vi "Initialize.vi"(8 "error in (no error)":errorcluster, 11 "HSDIO in":refnum<class "HSDIO.lvclass">) -> (0 "error out":errorcluster, 3 "HSDIO out":refnum<class "HSDIO.lvclass">)   [LabVIEW 2013, in "HSDIO.lvclass"]
uses:
  HSDIO.lvclass
  HSDIO.lvclass/HSDIO.ctl
  <instrlib>/niHSDIO/niHSDIO.llb/niHSDIO_ctl Sample Clock Source Values (ComboBox).ctl
  <instrlib>/niHSDIO/niHSDIO.llb/niHSDIO_ctl Generation Mode Values (Ring).ctl
  Globals.vi
  <instrlib>/niHSDIO/niHSDIO.llb/niHSDIO Configure Initial State (String).vi
  <instrlib>/niHSDIO/niHSDIO.llb/niHSDIO Configure Idle State (String).vi
  <instrlib>/niHSDIO/niHSDIO.llb/niHSDIO Configure Digital Edge Script Trigger.vi
  <instrlib>/niHSDIO/niHSDIO.llb/niHSDIO Configure Digital Level Script Trigger.vi
  <instrlib>/niHSDIO/niHSDIO.llb/niHSDIO Configure Digital Edge Start Trigger.vi
panel:
  out "HSDIO Settings.Idle State":string
  out "HSDIO Settings.Inital State":string
  out "HSDIO Status.Channel List":string
  out "instrument handle out":refnum<k15>
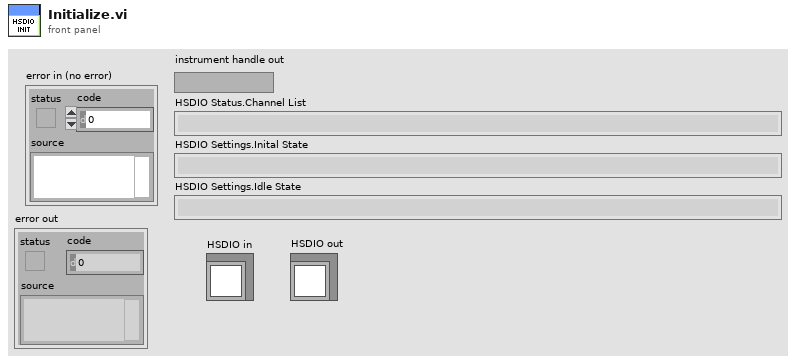
[diagram p1: front panel]
types:
  T1 = typedef "niHSDIO_ctl Sample Clock Source Values (ComboBox).ctl" = string
  T2 = typedef "niHSDIO_ctl Generation Mode Values (Ring).ctl" = i32
  T3 = typedef "niHSDIO_ctl Trigger Source Values (Ring).ctl" = string
  T4 = typedef "niHSDIO_ctl Trigger DigEdge - Edge Values (Ring).ctl" = i32
  T5 = cluster{"Wait for start trigger?":bool, "source (PFI 0)":T3, "edge (rising)":T4, "description":string}
  T6 = typedef "niHSDIO_ctl Trigger Script - trigID Values (Ring).ctl" = string
  T7 = typedef "niHSDIO_ctl Trigger DigLvl - Level Values (Ring).ctl" = i32
  T8 = cluster{"trigger id (script trigger 0)":T6, "source (PFI 0)":T3, "Trigger Type":enum32{"Edge", "Level"}, "edge":T4, "level":T7}[]
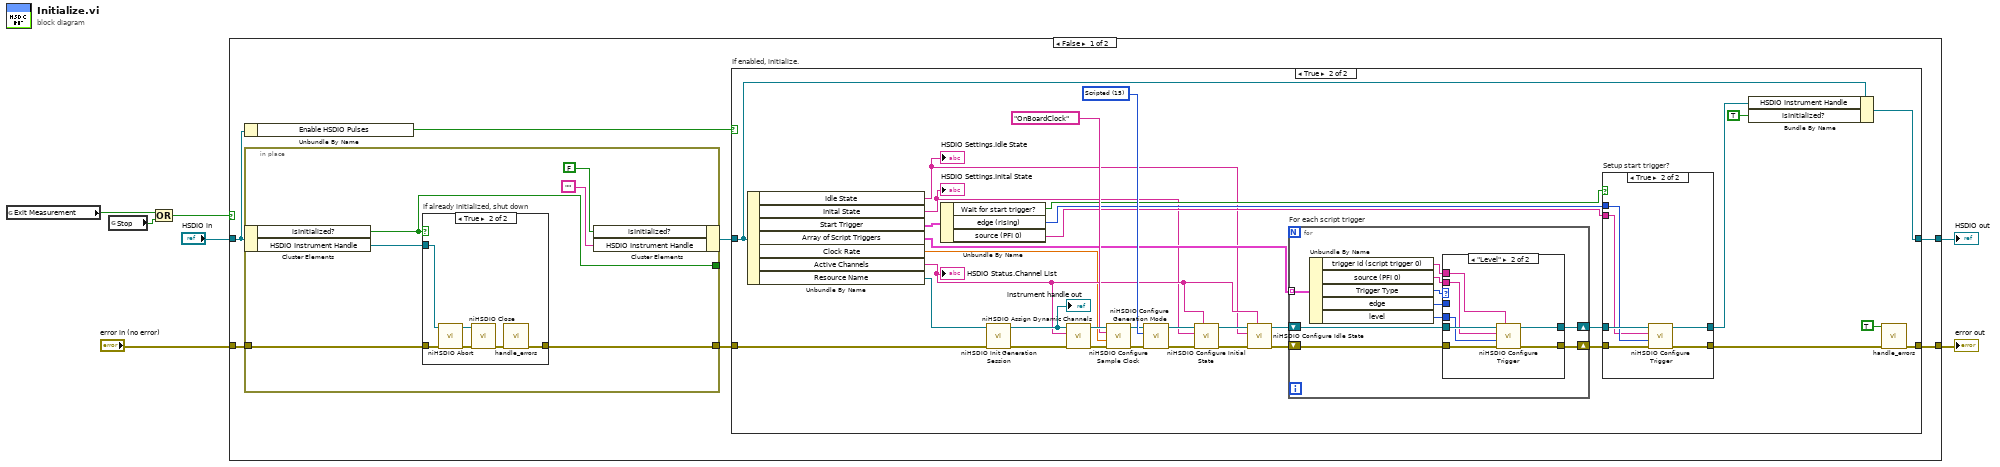
[diagram p0: block diagram]
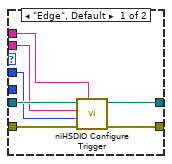
[diagram p4: hidden frame]
diagram:
  n1 = global read "Globals.vi" "Exit Measurement"() -> (w4:bool)
  n2 = global read "Globals.vi" "Stop"() -> (w3:bool)
  n3 = Or(x=w4, y=w3) -> (x .or. y?=w2:bool)
  n4 = case shown="False" w2 {
    tunnel: [w8 w96] -> w7
    tunnel: [w13 w97] -> w5
    tunnel: "HSDIO in" -> [w12 w97]
    tunnel: "error in (no error)" -> [w10 w96]
    frame False {
      n5 = Unbundle By Name(w12) -> ("Enable HSDIO Pulses"=w14:bool)
      n6 = in-place {
        in-place-border: [w17] -> _
        in-place-border: w10 -> [w20]
        in-place-border: [w19] -> w9
        n7 = in-place-cluster #1(w12) -> ("isInitialized?"=w17:bool, "HSDIO Instrument Handle"=w18:refnum<k15>)
        n8 = case "if already initialized, shut down" shown="True" w17 {
          tunnel: w20 -> [w21 w26]
          tunnel: [w21 w23] -> w19
          tunnel: w18 -> [_ w22]
          frame False {
          }
          frame True {
            n9 = call <instrlib>:"niHSDIO Abort.vi"("error in (no error)"=w26, "instrument handle"=w22) -> ("error out"=w25:errorcluster, "instrument handle out"=w27:refnum<k15>)  [unwired: 8 in]
            n10 = call <instrlib>:"niHSDIO Close.vi"("error in (no error)"=w25, "instrument handle"=w27) -> ("error out"=w24:errorcluster)  [unwired: 9 in]
            n11 = call "handle_errors.vi"("error in (no error)"=w24) -> ("error out"=w23:errorcluster)  [unwired: 14 in]
          }
        }
        n12 = in-place-cluster #1("isInitialized?"=FALSE, "HSDIO Instrument Handle"="") -> (w11:refnum<class "HSDIO.lvclass">)
      }
      n13 = case "If enabled, initialize." shown="True" w14 {
        tunnel: [w29 w35] -> w8
        tunnel: w11 -> [w28 w38]
        tunnel: [w28 w41] -> w13
        tunnel: w9 -> [w29 w37]
        frame False {
        }
        frame True {
          w56 = T2 15 items=["Waveform"=14, "Scripted"=15] ("generation mode (waveform)")
          n14 = Unbundle By Name(w38) -> ("Idle State"=w39:string, "Inital State"=w40:string, "Start Trigger"=w50:T5, "Array of Script Triggers"=w46:T8, "Clock Rate"=w51:dbl, "Active Channels"=w52:string, "Resource Name"=w53:refnum<k15>)
          "HSDIO Status.Channel List" <- w52
          "HSDIO Settings.Inital State" <- w40
          "HSDIO Settings.Idle State" <- w39
          n15 = Unbundle By Name(w50) -> ("Wait for start trigger?"=w47:bool, "edge (rising)"=w49:T4, "source (PFI 0)"=w48:T3)
          n16 = call <instrlib>:"niHSDIO Init Generation Session.vi"("error in (no error)"=w37, "resource name"=w53) -> ("error out"=w58:errorcluster, "instrument handle out"=w63:refnum<k15>)  [unwired: 8 in]
          "instrument handle out" <- w63
          n17 = call <instrlib>:"niHSDIO Assign Dynamic Channels.vi"("error in (no error)"=w58, "channel list (all:\"\")"=w52, "instrument handle"=w63) -> ("error out"=w57:errorcluster, "instrument handle out"=w62:refnum<k15>)  [unwired: 7 in]
          n18 = call <instrlib>:"niHSDIO Configure Sample Clock.vi"("error in (no error)"=w57, "clock rate (50MHz)"=w51, "clock source (on board clock)"=T1 "OnBoardClock", "instrument handle"=w62) -> ("error out"=w32:errorcluster, "instrument handle out"=w33:refnum<k15>)  [unwired: 6 in]
          n19 = call <instrlib>:"niHSDIO Configure Generation Mode.vi"("error in (no error)"=w32, "generation mode (waveform)"=w56, "instrument handle"=w33) -> ("error out"=w55:errorcluster, "instrument handle out"=w54:refnum<k15>)  [unwired: 7 in]
          n20 = call-poly <instrlib>:"niHSDIO Configure Initial State.vi"("channel list"=w52, "error in (no error)"=w55, "initial state"=w40, "instrument handle"=w54) -> ("error out"=w59:errorcluster, "instrument handle out"=w60:refnum<k15>)  [unwired: 6 in]
          n21 = call-poly <instrlib>:"niHSDIO Configure Idle State.vi"("channel list"=w52, "error in (no error)"=w59, "idle state"=w39, "instrument handle"=w60) -> ("error out"=w45:errorcluster, "instrument handle out"=w44:refnum<k15>)  [unwired: 6 in]
          n22 = for "For each script trigger" {
            tunnel: w46 -> [w73] mode=indexing
            shift-right: [w71] -> w43
            shift-left: w45 -> [w72]
            shift-right: [w70] -> w42
            shift-left: w44 -> [w69]
            n23 = Unbundle By Name(w73) -> ("trigger id (script trigger 0)"=w68:T6, "source (PFI 0)"=w67:T3, "Trigger Type"=w66:enum32{"Edge", "Level"}, "edge"=w65:T4, "level"=w64:T7)
            n24 = case shown="\"Level\"" w66 {
              tunnel: w72 -> [w80 w87]
              tunnel: [w79 w86] -> w71
              tunnel: [w78 w84] -> w70
              tunnel: w69 -> [w77 w85]
              tunnel: w68 -> [w76 w83]
              tunnel: w67 -> [w75 w82]
              tunnel: w65 -> [w74 _]
              tunnel: w64 -> [_ w81]
              frame "Edge", Default {
                n25 = call-poly <instrlib>:"niHSDIO Configure Trigger.vi"("trigger id (script trigger 0)"=w76, "error in (no error)"=w80, "edge (rising)"=w74, "source (PFI 0)"=w75, "instrument handle"=w77) -> ("error out"=w79:errorcluster, "instrument handle out"=w78:refnum<k15>)  [unwired: 5 in]
              }
              frame "Level" {
                n26 = call-poly <instrlib>:"niHSDIO Configure Trigger.vi"("trigger id (script trigger 0)"=w83, "error in (no error)"=w87, "trigger when (high)"=w81, "source (PFI 0)"=w82, "instrument handle"=w85) -> ("error out"=w86:errorcluster, "instrument handle out"=w84:refnum<k15>)  [unwired: 5 in]
              }
            }
          }
          n27 = case "Setup start trigger?" shown="True" w47 {
            tunnel: w43 -> [w89 w95]
            tunnel: [w89 w94] -> w30
            tunnel: w42 -> [w88 w93]
            tunnel: [w88 w92] -> w31
            tunnel: w49 -> [_ w91]
            tunnel: w48 -> [_ w90]
            frame False {
            }
            frame True {
              n28 = call-poly <instrlib>:"niHSDIO Configure Trigger.vi"("error in (no error)"=w95, "edge (rising)"=w91, "source (PFI 0)"=w90, "instrument handle"=w93) -> ("error out"=w94:errorcluster, "instrument handle out"=w92:refnum<k15>)  [unwired: 6 in]
            }
          }
          n29 = Bundle By Name(cluster=w38, "HSDIO Instrument Handle"=w31, "isInitialized?"=TRUE) -> (w41:refnum<class "HSDIO.lvclass">)
          n30 = call "handle_errors.vi"("Exit Operation"=TRUE ("Exit Measurement"), "error in (no error)"=w30) -> ("error out"=w35:errorcluster)  [unwired: 13 in]
        }
      }
    }
    frame True {
    }
  }
  "error out" <- w7
  "HSDIO out" <- w5
